vi "Date 2 Sortable Date.vi"(3 "Date String":string="May/02/18 15:50:37") -> (1 "Sortable Date":string)   [LabVIEW 2013]
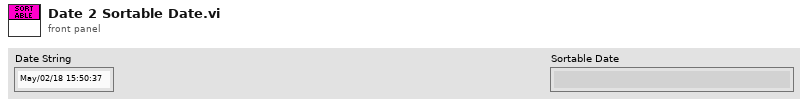
[diagram p1: front panel]
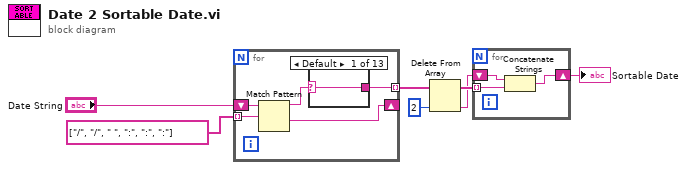
[diagram p0: block diagram]
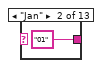
[diagram p2: hidden frame]
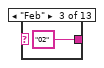
[diagram p3: hidden frame]
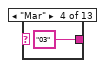
[diagram p4: hidden frame]
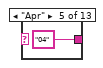
[diagram p5: hidden frame]
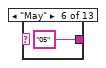
[diagram p6: hidden frame]
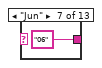
[diagram p7: hidden frame]
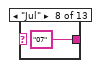
[diagram p8: hidden frame]
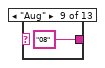
[diagram p9: hidden frame]
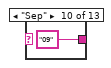
[diagram p10: hidden frame]
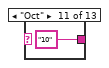
[diagram p11: hidden frame]
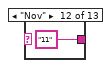
[diagram p12: hidden frame]
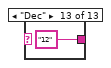
[diagram p13: hidden frame]
diagram:
  n1 = for {
    shift-right: [w11] -> _
    shift-left: "Date String" -> [w12]
    tunnel: [w8] -> w5 mode=indexing
    tunnel: string[] ["/", "/", " ", ":", ":", ":"] -> [w10] mode=indexing
    n2 = Match Pattern(string=w12, regular expression=w10) -> (before substring=w9:string, after substring=w11:string)  [unwired: 1 in, 2 out]
    n3 = case shown="Default" w9 {
      selector: w9 -> [w13 _ _ _ _ _ _ _ _ _ _ _ _]
      tunnel: [w13 "01" "02" "03" "04" "05" "06" "07" "08" "09" "10" "11" "12"] -> w8
      frame Default {
      }
      frame "Jan" {
      }
      frame "Feb" {
      }
      frame "Mar" {
      }
      frame "Apr" {
      }
      frame "May" {
      }
      frame "Jun" {
      }
      frame "Jul" {
      }
      frame "Aug" {
      }
      frame "Sep" {
      }
      frame "Oct" {
      }
      frame "Nov" {
      }
      frame "Dec" {
      }
    }
  }
  n4 = Delete From Array(array=w5, index=2) -> (deleted portion=w1:string, array with subset deleted=w3:string[])  [unwired: 1 in]
  n5 = for {
    tunnel: w3 -> [w27] mode=indexing
    shift-right: [w26] -> w2
    shift-left: w1 -> [w28]
    n6 = Concatenate Strings(w28, w27) -> (w26:string)
  }
  "Sortable Date" <- w2
